vi "Measure.vi"(8 "error in (no error)":errorcluster, 9 "measurement configuration":variant, 10 "measure call context in":refnum<class "Measure Call Context.lvclass">, 11 "measurement plugin in":refnum<class "Ni-Scope-Multirecords.lvclass">) -> (0 "error out":errorcluster, 1 "measurement results":variant, 2 "measure call context out":refnum<class "Measure Call Context.lvclass">, 3 "measurement plugin out":refnum<class "Ni-Scope-Multirecords.lvclass">)   [LabVIEW 2025, in "Ni-Scope-Multirecords.lvclass"]
uses:
  Ni-Scope-Multirecords.lvclass
  <vilib>/Plug-In SDKs/Measurements/Measure Call Context/Measure Call Context.lvclass
  Measurement Configuration.ctl
  Ni-Scope-Multirecords.lvclass/Ni-Scope-Multirecords.ctl
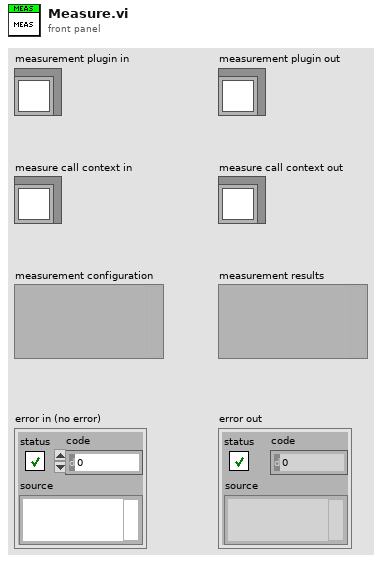
[diagram p1: front panel]
types:
  T1 = typedef "Ni-Scope-Multirecords.lvclass/Measurement Configuration.ctl" = cluster{"Resource Name(s)":string[], "Number Of Records":i32, "Timeout (s)":dbl, "Configuration File Path":string, "Delay Mode":string, "Horizontal Position":dbl, "Length Unit":string, "Record Length":dbl, "Stream To File Path":string}
  T2 = typedef "Ni-Scope-Multirecords.lvclass/Measurement Results.ctl" = cluster{"RelativeInitialX":dbl[], "xIncrement":dbl[], "Wfm":dbl[][], "Plot Names":string[], "Actual Sample Rate":dbl, "Actual Record Duration":dbl, "Actual Record Length":dbl}
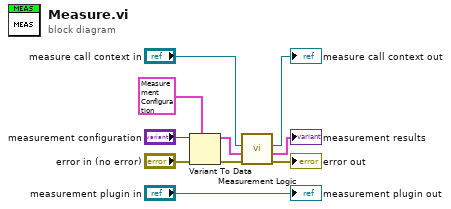
[diagram p0: block diagram]
diagram:
  n1 = Variant To Data(error in="error in (no error)", type=T1 {"Resource Name(s)"=[], "Number Of Records"=32, "Timeout (s)"=1.2, "Configuration File Path"="", "Delay Mode"="On", "Horizontal Position"=0.0, "Length Unit"="Percentage", "Record Length"=100.0, "Stream To File Path"=""} ("measurement configuration"), Variant="measurement configuration") -> (data=w1:T1, error out=w7:errorcluster)
  n2 = call "Measurement Logic.vi"("error in"=w7, "measurement configuration"=w1, "measure call context in"="measure call context in") -> ("error out"=→"error out":errorcluster, "measurement results"=→"measurement results":T2, "measure call context out"=→"measure call context out":refnum<class "Measure Call Context.lvclass">)  [unwired: 6 in]
  "measurement plugin out" <- "measurement plugin in"
